vi "TEST - Trim Whitespace__og.vi"(8 "error in (no error)":errorcluster) -> (0 "error out":errorcluster, 2 "pass":bool)   [LabVIEW 2013]
uses:
  source/library/Trim Whitespace/Trim Whitespace (String).vi
panel:
  out "Failures":T1(array[cluster])
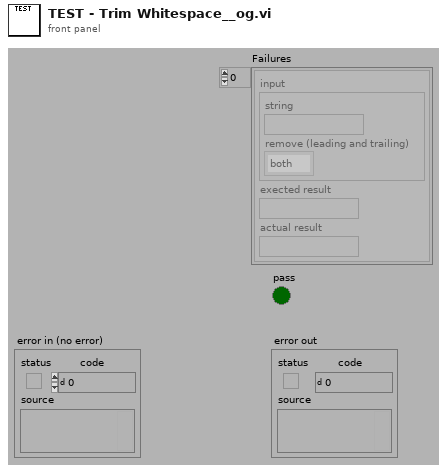
[diagram p1: front panel]
types:
  T1 = cluster{"input":cluster{"string":string, "remove (leading and trailing)":enum16{"leading", "trailing", "both"}}, "exected result":string, "actual result":string}[]
  T2 = cluster{"input":cluster{"string":string, "remove":enum16{"leading", "trailing", "both"}}, "exected result":string, "actual result":string}[]
  T3 = cluster{"input":cluster{"string":string, "remove":enum16{"leading", "trailing", "both"}}, "exected result":string, "actual result":string}
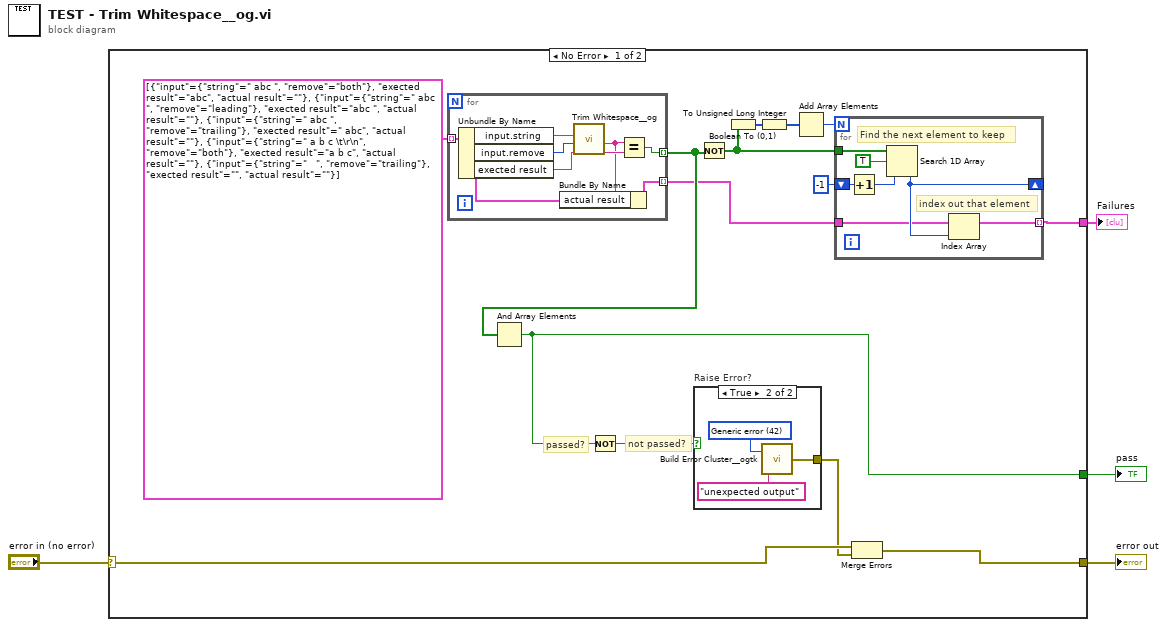
[diagram p0: block diagram]
diagram:
  n1 = case shown="No Error" "error in (no error)" {
    selector: "error in (no error)" -> [w18 w36]
    tunnel: [w13 _] -> w4
    tunnel: [w17 w36] -> w2
    tunnel: [w5 _] -> w1
    frame No Error {
      # "not passed?"
      # "passed?"
      n2 = for {
        tunnel: T2 [{"input"={"string"=" abc ", "remove"=enum."both"}, "exected result"="abc", "actual result"=""}, {"input"={"string"=" abc ", "remove"=enum."leading"}, "exected result"="abc ", "actual result"=""}, {"input"={"string"=" abc ", "remove"=enum."trailing"}, "exected result"=" abc", "actual result"=""}, {"input"={"string"=" a b c \t\r\n", "remove"=enum."both"}, "exected result"="a b c", "actual result"=""}, {"input"={"string"="   ", "remove"=enum."trailing"}, "exected result"="", "actual result"=""}] -> [w29] mode=indexing
        tunnel: [w32] -> w7 mode=indexing
        tunnel: [w30] -> w6 mode=indexing
        n3 = Unbundle By Name(w29) -> ("input.string"=w28:string, "input.remove"=w27:enum16{"leading", "trailing", "both"}, "exected result"=w31:string)
        n4 = call-poly "Trim Whitespace__og.vi"("Remove (leading and trailing)"=w27, "String in"=w28) -> ("String out"=w26:string)  [unwired: 5 in]
        n5 = Bundle By Name(cluster=w29, "actual result"=w26) -> (w30:T3)
        n6 = Equal?(x=w26, y=w31) -> (x = y?=w32:bool)
      }
      n7 = And Array Elements(Boolean array=w7) -> (logical AND=w13:bool)
      n8 = Not(x=w13) -> (.not. x?=w15:bool)
      n9 = case "Raise Error?" shown="True" w15 {
        tunnel: [_ w33] -> w16
        frame False {
        }
        frame True {
          w34 = 42 items=["No error", "Argument error", "Memory is full", "Out of zone", "End of file", "File already open", "Generic file I/O error", "File not found", "File permission error", "Disk is full", "Duplicate path", "Too many files open", "System feature not enabled", "Resource file not found", "Cannot add resource", "Resource not found", "Image not found", "Image memory error", "Pen does not exist", "Config type invalid", "Config token not found", "Config parse error", "Config memory error", "Bad external code format", "Bad external code offset", "External code not present", "Null window", "Destroy window error", "Null menu", "Print aborted", "Bad print record", "Print driver error", "Windows error during printing", "Memory error during printing", "Print dialog error", "Generic print error", "Invalid device refnum", "Device not found", "Device parameter error", "Device unit error", "Cannot open device", "Device call aborted", "Generic error", "Cancelled by user", "Object ID too low", "Object ID too high", "Object not in heap", "Unknown heap", "Unknown object (invalid DefProc)", "Unknown object (DefProc not in table)", "Message out of range", "Invalid (null) method", "Unknown message", "Manager call not supported", "Bad address", "Network operation in progress", "Network operation timed out", "Connection is busy", "Network attribute not supported", "Network error", "Address in use", "System out of memory", "Connection aborted", "Connection refused", "Not connected", "Already connected", "Connection closed", "Initialization error (interapplication manager)", "Bad occurrence", "Wait on unbound occurrence handler", "Occurrence queue overflow", "Datalog type conflict", "Unused", "Unrecognized type (interapplication manager)", "Memory corrupt", "Failed to make temporary DLL", "Old CIN version", "Drag socket not found", "Failed to load drop-object", "Failed to register OLE object", "Failed to release OLE object", "Format specifier type mismatch", "Unknown format specifier", "Too few format specifiers", "Too many format specifiers", "Scan failed", "Newer CIN version", "Error converting to variant", "Runtime menu error", "Password tampered", "Variant attribute not found", "Incompatible variant data type", "Event data is not available", "Event Store is not present", "Occurrence is not found", "Event Queue is not created", "Event info is not available", "Refnum passed is NULL", "Error retrieving Class GUID", "Error retrieving CoClass GUID", "Error retrieving TypeLib GUID.", "Bad built application magic bytes.", "Specific driver is different from the specific driver associated with the Logical Name.", "There is no session opened to the class driver.", "Max Error", "MAX - Error with config objects", "MAX - Error loading configuration", "MAX - Group not supported"]
          n10 = call <userlib>:"Build Error Cluster__ogtk.vi"("String to Prepend to source (\"\")"="unexpected output" ("String to Prepend to source (\"\")"), "code"=w34) -> ("error out"=w33:errorcluster)
        }
      }
      n11 = Not(x=w7) -> (.not. x?=w9:bool[])
      n12 = Boolean To (0,1)(Boolean=w9) -> (0, 1=w10:i16[])
      n13 = To Unsigned Long Integer(number=w10) -> (unsigned 32bit integer=w8:u32[])
      n14 = Add Array Elements(numeric array=w8) -> (sum=w11:u32)
      n15 = for {
        N: w11 -> [_]
        tunnel: w6 -> [w21]
        tunnel: w9 -> [w25]
        shift-right: [w22] -> _
        shift-left: -1 ("start index (0)") -> [w23]
        tunnel: [w20] -> w5 mode=indexing
        # "index out that element"
        # "Find the next element to keep"
        n16 = Increment(x=w23) -> (x+1=w19:i32)
        n17 = Search 1D Array(1D array=w25, element=TRUE, start index (0)=w19) -> (index of element=w22:i32)
        n18 = Index Array(array=w21, index=w22) -> (element=w20:T3)
      }
      n19 = Merge Errors(w18, w16) -> (w17:errorcluster)
    }
    frame Error {
    }
  }
  "pass" <- w4
  "error out" <- w2
  "Failures" <- w1
